vi "COM_Prepare Eigenvalues.vi"(10 "dt":dbl, 11 "Eigenvalues":cdb[](array[numeric])) -> (0 "error":i32, 3 "Modes OUT":T1(array[cluster]))   [LabVIEW 2017, in "AppPlugins.lvlib" / "EraPlugin.lvclass"]
uses:
  EraPlugin.lvclass
  <vilib>/Analysis/NI_AALPro.lvlib
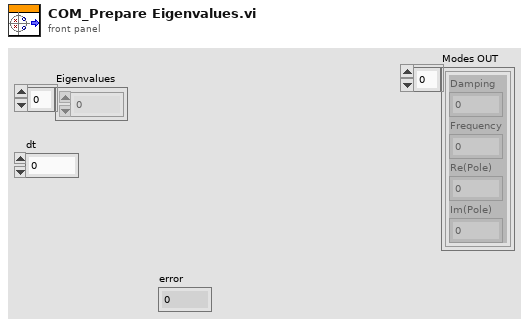
[diagram p1: front panel]
types:
  T1 = cluster{"Damping":dbl, "Frequency":dbl, "Re(Pole)":dbl, "Im(Pole)":dbl}[]
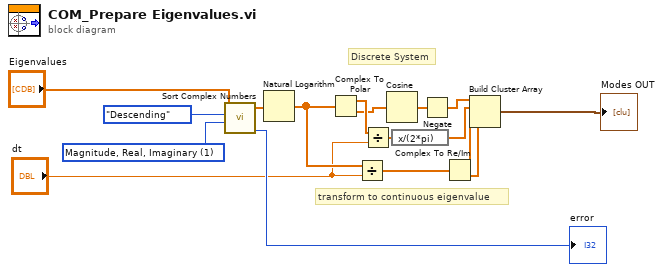
[diagram p0: block diagram]
diagram:
  w9 = u16 1 items=["Real, Imaginary", "Magnitude, Real, Imaginary", "Magnitude, Phase Angle"] ("method")
  # "transform to continuous eigenvalue"
  # "Discrete System"
  n1 = call <vilib>:"Sort Complex Numbers.vi"("method"=w9, "order"=enum16{"Ascending", "Descending"}."Descending", "Complex Numbers"="Eigenvalues") -> ("error"=→"error":i32, "Sorted Complex Numbers"=w10:cdb[])  [unwired: 6 in, 1 out]
  n2 = Natural Logarithm(1:w10) -> (0:w4:cdb[])
  n3 = Complex To Polar(r * e^(i*theta)=w4) -> (r=w16:dbl[], theta=w7:dbl[])
  n4 = Divide(x=w4, y="dt") -> (x/y=w2:cdb[])
  n5 = Divide(x=w16, y="dt") -> (x/y=w8:dbl[])
  n6 = Cosine(x=w7) -> (cos(x)=w6:dbl[])
  n7 = expression code="x/(2*pi)"(w8) -> (w13:dbl[])
  n8 = Negate(x=w6) -> (-x=w15:dbl[])
  n9 = Complex To Re/Im(x + iy=w2) -> (x=w11:dbl[], y=w12:dbl[])
  n10 = Build Cluster Array(w15, w13, w11, w12) -> (→"Modes OUT":cluster{"Numeric":dbl, dbl, dbl, dbl}[])
